vi "CMD_Run.vi"(1 "Line":string) -> (0 "Done":bool)   [LabVIEW 2015]
panel:
  in  "Parameters":i32[](array[numeric])=[1, 1, 1, 1]
  in  "Subcommands":string[](array[string])=["motor", "at", "for", "until"]
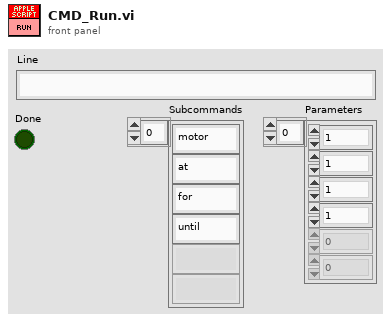
[diagram p1: front panel]
types:
  T1 = typedef "WPI_MotorControlDeviceRef.ctl" = cluster{"DeviceStatus":errorcluster, "Type":enum16{"PWM", "CAN"}, "PWM":cluster{"Digital Module":T2, "PWM Channel":T3, "DeadBand":T4}, "CAN":cluster{"Device Number":u8, "Control Mode":T5, "Semaphore":T6, "Max Vout":dbl}, "Invert":bool, "TransformRef":T7, "InvTransformRef":T7}
  T2 = typedef "FPGA_TypedefDigitalModule.ctl" = enum16{"Digital Module 1", "Digital Module 2"}
  T3 = typedef "FPGA_DIOPWMChannel.ctl" = enum8{"PWM 1", "PWM 2", "PWM 3", "PWM 4", "PWM 5", "PWM 6", "PWM 7", "PWM 8", "PWM 9", "PWM 10", "Invalid"}
  T4 = typedef "WPI_PWMDeadband.ctl" = cluster{"Name":string, "maxPositivePwm":i32, "minPositivePwm":i32, "centerPwm":i32, "maxNegativePwm":i32, "minNegativePwm":i32, "angularRange":u16}
  T5 = typedef "WPI_CANJaguar_ControlMode.ctl" = enum8{"Percent VBus", "Current", "Speed", "Position", "Voltage"}
  T6 = typedef "Semaphore RefNum" = refnum<k1>
  T7 = typedef "WPI_PWMTransform_ConPane.ctl" = refnum<vi>
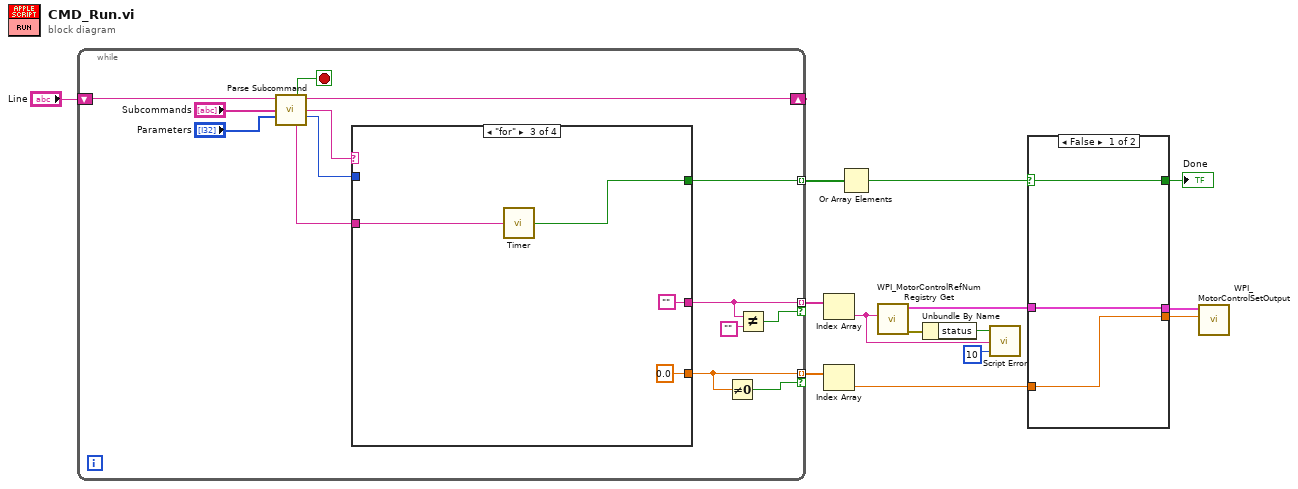
[diagram p0: block diagram]
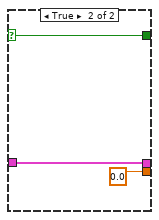
[diagram p2: hidden frame]
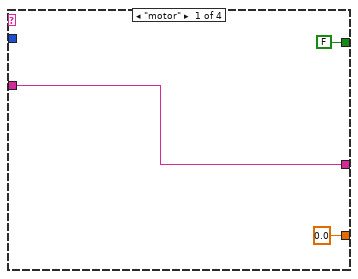
[diagram p3: hidden frame]
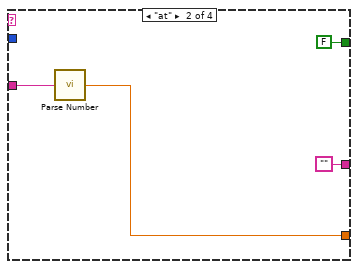
[diagram p4: hidden frame]
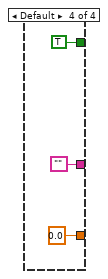
[diagram p5: hidden frame]
diagram:
  n1 = while {
    shift-right: [w25] -> _
    shift-left: "Line" -> [w28]
    tunnel: [w20] -> w13 mode=indexing
    tunnel: [w19] -> w12 mode=indexing if=w17
    tunnel: [w16] -> w11 mode=indexing if=w15
    stop <- w24 stop-if-true
    n2 = call "Parse Subcommand.vi"("Text In"=w28, "Subcommands"="Subcommands", "Parameters"="Parameters") -> ("Done"=w24:bool, "Text Out"=w25:string, "Subcommand"=w23:string, "# of Parameters"=w22:i32, "Parameter 1"=w21:string)  [unwired: 6 in, 2 out]
    n3 = case shown="\"for\"" w23 {
      tunnel: w22 -> [_ _ _ _]
      tunnel: w21 -> [w29 w35 w39 _]
      tunnel: [FALSE FALSE ("Value") w36 TRUE ("Value")] -> w20
      tunnel: [w29 "" "" ""] -> w19
      tunnel: [0.0 ("Number") w32 0.0 ("Number") 0.0 ("Number")] -> w16
      frame "motor" {
      }
      frame "at" {
        n4 = call "Parse Number.vi"("String"=w35) -> ("Number"=w32:dbl)
      }
      frame "for" {
        n5 = call "Timer.vi"("Seconds (string)"=w39) -> ("Done"=w36:bool)
      }
      frame Default {
      }
    }
    n6 = Not Equal To 0?(x=w16) -> (x != 0?=w15:bool)
    n7 = Not Equal?(x=w19, y="") -> (x != y?=w17:bool)
  }
  n8 = Index Array(array=w12) -> (element=w1:string)  [unwired: 1 in]
  n9 = Index Array(array=w11) -> (element=w6:dbl)  [unwired: 1 in]
  n10 = Or Array Elements(Boolean array=w13) -> (logical OR=w10:bool)
  n11 = call <vilib>:"WPI_MotorControlRefNum Registry Get.vi"("refnum name"=w1) -> ("error out"=w4:errorcluster, "MotorControlDevRef"=w8:T1)  [unwired: 9 in]
  n12 = Unbundle By Name(w4) -> ("status"=w2:bool)
  n13 = call "Script Error.vi"("Error?"=w2, "Error Details"=w1, "Error Code"=10) -> ()  [unwired: 2 in, 1 out]
  n14 = case shown="False" w10 {
    selector: w10 -> [w45 w48]
    tunnel: [w45 w48] -> w9
    tunnel: w8 -> [w44 w47]
    tunnel: [w44 w47] -> w7
    tunnel: w6 -> [w43 _]
    tunnel: [w43 0.0] -> w5
    frame False {
    }
    frame True {
    }
  }
  "Done" <- w9
  n15 = call <vilib>:"WPI_MotorControlSetOutput.vi"("Output"=w5, "MotorControlDevRef"=w7) -> ()  [unwired: 7 in, 3 out]
